vi "GSI-HVSwitch2.contents.vi"() -> ()   [LabVIEW 2014, in "GSI-HVSwitch2.lvlib"]
doc: "Contains \"all\" VIs. Required for building applications."
uses:
  GSI-HVSwitch2.lvlib
panel:
  out "error out":errorcluster
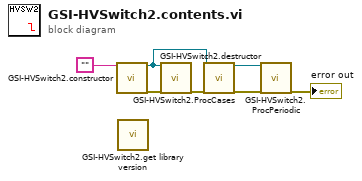
[diagram p0: block diagram]
diagram:
  n1 = call "GSI-HVSwitch2.constructor.vi"("name"="") -> ("i ref out"=w5:refnum<vi>, "error out"=w4:errorcluster)  [unwired: 16 in, 1 out]
  n2 = call "GSI-HVSwitch2.get library version.vi"() -> ()  [unwired: 1 in, 1 out]
  n3 = call "GSI-HVSwitch2.destructor.vi"("i ref in"=w5, "error in (no error)"=w4) -> ("error out"=w3:errorcluster)  [unwired: 17 in]
  n4 = call "GSI-HVSwitch2.ProcCases.vi"("i ref in"=w5, "error in (no error)"=w3) -> ("i ref out"=w7:refnum<vi>, "error out"=w2:errorcluster)  [unwired: 15 in, 1 out]
  n5 = call "GSI-HVSwitch2.ProcPeriodic.vi"("i ref in"=w7, "error in (no error)"=w2) -> ("error out"=→"error out":errorcluster)  [unwired: 15 in, 2 out]
